vi "Get Cells in Path.vi"(8 "error in (no error)":errorcluster, 10 "path references":refnum<data-value>[](array[refnum]), 11 "map reference in":refnum<data-value>) -> (0 "error out":errorcluster, 1 "y coordinates":i32[](array[numeric]), 2 "x coordinates":i32[](array[numeric]), 3 "map reference out":refnum<data-value>)   [LabVIEW 2017, in "NI_Robotics_OccupancyGridWorldMap.lvclass"]
doc: "Returns the cell coordinates of the points along a path through an occupancy grid map."
uses:
  <vilib>/robotics/Navigation/shared/WorldMap/OccupancyGridWorldMap/NI_Robotics_OccupancyGridWorldMap.lvclass
  <vilib>/robotics/Navigation/shared/MapNode/AbstractAstarNode/NI_Robotics_AbstractAstarNode.lvclass
  <vilib>/robotics/Navigation/shared/MapNode/OccupancyGridNode/NI_Robotics_OccupancyGridMapNode.lvclass
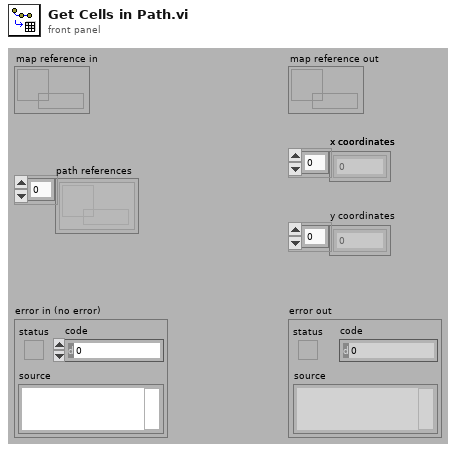
[diagram p1: front panel]
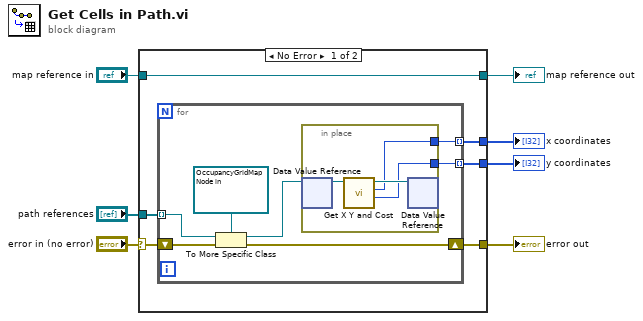
[diagram p0: block diagram]
diagram:
  n1 = case shown="No Error" "error in (no error)" {
    selector: "error in (no error)" -> [w12 w25]
    tunnel: "path references" -> [w13 _]
    tunnel: [w11 w26] -> w4
    tunnel: "map reference in" -> [w11 w26]
    tunnel: [w10 _] -> w3
    tunnel: [w9 _] -> w2
    tunnel: [w8 w25] -> w1
    frame No Error {
      n2 = for {
        tunnel: w13 -> [w19] mode=indexing
        shift-right: [w15] -> w8
        shift-left: w12 -> [w20]
        tunnel: [w17] -> w10 mode=indexing
        tunnel: [w16] -> w9 mode=indexing
        n3 = To More Specific Class(target class=refnum<data-value> refnum ("cell reference"), reference=w19, error in=w20) -> (specific class reference=w18:refnum<data-value>, error out=w15:errorcluster)
        n4 = in-place {
          in-place-border: [w22] -> w17
          in-place-border: [w21] -> w16
          n5 = in-place-dvr #1(w18) -> (w24:refnum<class "NI_Robotics_OccupancyGridMapNode.lvclass">)  [unwired: 1 out]
          n6 = call-dynamic "Get X Y and Cost.vi"("OccupancyGridMapNode in"=w24) -> ("y"=w21:i32, "x"=w22:i32, "OccupancyGridMapNode out"=w23:refnum<class "NI_Robotics_OccupancyGridMapNode.lvclass">)  [unwired: 7 in, 1 out]
          n7 = in-place-dvr #1(w23) -> ()  [unwired: 2 out]
        }
      }
    }
    frame Error {
    }
  }
  "map reference out" <- w4
  "error out" <- w1
  "x coordinates" <- w3
  "y coordinates" <- w2
